vi "Load Sequence.vi"(8 "Error In":errorcluster, 10 "Selected Path":path, 11 "CS++SeqEditor in":refnum<class "CS++SeqEditor.lvclass">) -> (0 "Error Out":errorcluster, 3 "CS++SeqEditor out":refnum<class "CS++SeqEditor.lvclass">)   [LabVIEW 2016, in "CS++SeqEditor.lvlib" / "CS++SeqEditor.lvclass"]
doc: "load sequence from file."
uses:
  CS++SeqEditor.lvclass
  CS++SeqEditor.lvclass/CS++SeqEditor.ctl
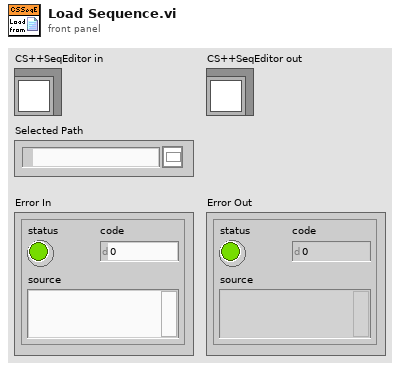
[diagram p1: front panel]
types:
  T1 = enum16{"open", "replace", "create", "open or create", "replace or create", "replace or create with confirmation"}
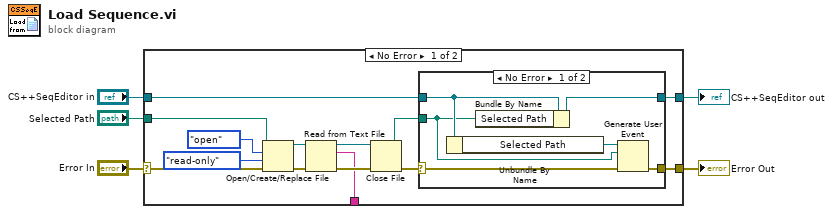
[diagram p0: block diagram]
diagram:
  n1 = case shown="No Error" "Error In" {
    selector: "Error In" -> [w13 w29]
    tunnel: [w9 w29] -> w4
    tunnel: [w18 w28] -> w2
    tunnel: "CS++SeqEditor in" -> [w19 w28]
    tunnel: "Selected Path" -> [w7 _]
    tunnel: [w8 _] -> _
    frame No Error {
      n2 = Open/Create/Replace File(file path (use dialog)=w7, error in=w13, operation (0:open)=T1."open", access (0:read/write)=enum16{"read/write", "read-only", "write-only"}."read-only") -> (refnum out=w15:refnum<file>, error out=w14:errorcluster)  [unwired: 2 in, 1 out]
      n3 = Read from Text File(file (use dialog)=w15, error in=w14) -> (refnum out=w11:refnum<file>, text=w8:string, error out=w12:errorcluster)  [unwired: 2 in, 1 out]
      n4 = Close File(refnum=w11, error in=w12) -> (path=w6:path, error out=w10:errorcluster)
      n5 = case shown="No Error" w10 {
        selector: w10 -> [w21 w26]
        tunnel: w19 -> [w24 w27]
        tunnel: [w25 w27] -> w18
        tunnel: w6 -> [w22 _]
        tunnel: [w20 w26] -> w9
        frame No Error {
          n6 = Unbundle By Name(w24) -> ("Selected Path"=w23:refnum<user-event>)
          n7 = Bundle By Name(cluster=w24, "Selected Path"=w22) -> (w25:refnum<class "CS++SeqEditor.lvclass">)
          n8 = Generate User Event(user event=w23, event data cluster=w22, error in=w21) -> (error out=w20:errorcluster)  [unwired: 1 in, 1 out]
        }
        frame Error {
        }
      }
    }
    frame Error {
    }
  }
  "Error Out" <- w4
  "CS++SeqEditor out" <- w2
